vi "Propagate Theme To Nested Appearance Actors.vi"(8 "Error In":errorcluster, 11 "Appearance Actor in":refnum<class "Appearance Actor.lvclass">) -> (0 "Error Out":errorcluster, 3 "Appearance Actor out":refnum<class "Appearance Actor.lvclass">)   [LabVIEW 2021, in "Appearance Actor.lvlib" / "Appearance Actor.lvclass"]
doc: "Override this vi to send the Theme to nested Actors."
uses:
  Appearance Actor.lvclass
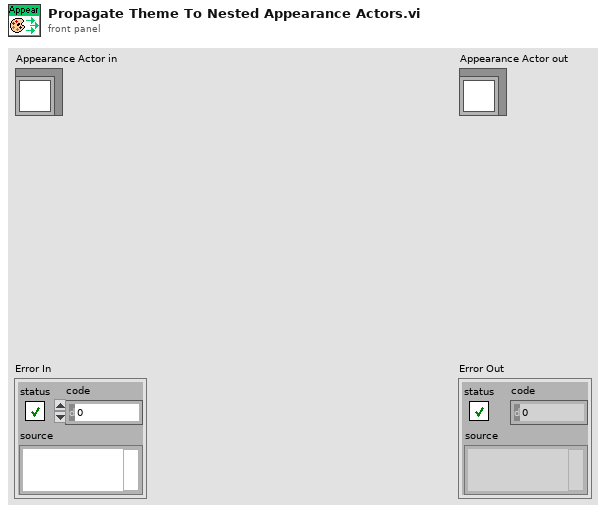
[diagram p1: front panel]
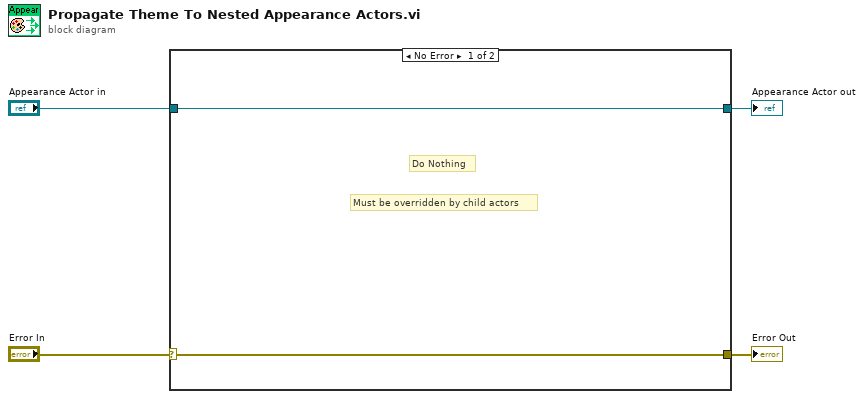
[diagram p0: block diagram]
diagram:
  n1 = case shown="No Error" "Error In" {
    selector: "Error In" -> [w6 w8]
    tunnel: [w6 w8] -> w3
    tunnel: [w5 w7] -> w1
    tunnel: "Appearance Actor in" -> [w5 w7]
    frame No Error {
      # "Must be overridden by child actors"
      # "Do Nothing"
    }
    frame Error {
    }
  }
  "Error Out" <- w3
  "Appearance Actor out" <- w1
